vi "Initialize.vi"(8 "error in":errorcluster, 11 "Plugin in":refnum<class "Sift Stream.lvclass">) -> (0 "error out":errorcluster, 3 "Plugin out":refnum<class "Sift Stream.lvclass">)   [LabVIEW 2024, in "Sift Stream.lvlib" / "Sift Stream.lvclass"]
uses:
  Sift Stream.lvclass
  Sift Stream.lvclass/Sift Stream.ctl
  <vilib>/FlexLogger/SDK/PluginSDK.lvlibp/PEFClasses/SDK/Plugin/Plugin.lvclass
  <vilib>/FlexLogger/SDK/PluginSDK.lvlibp/PEFClasses/SDK/Processing Element/Timing Method.ctl
  <vilib>/FlexLogger/SDK/PluginSDK.lvlibp/PEFClasses/SDK/Processing Element/Processing Element.lvclass
  <vilib>/FlexLogger/SDK/PluginSDK.lvlibp/PEFClasses/SDK/Processing Element/Timing Parameters.ctl
  <vilib>/FlexLogger/SDK/PluginSDK.lvlibp/PEFClasses/SDK/Plugin/ParameterAccess/Write String.vi
  <vilib>/FlexLogger/SDK/PluginSDK.lvlibp/PEFClasses/SDK/Plugin/ParameterAccess/Write DBL.vi
  <vilib>/FlexLogger/SDK/PluginSDK.lvlibp/PEFClasses/SDK/Plugin/ParameterAccess/Write N Channel.vi
  C:/Program Files/National Instruments/LabVIEW 2024/vi.lib/FlexLogger/SDK/PluginSDK.lvlibp/PEFClasses/SDK/Plugin/Plugin.lvclass
  C:/Program Files/National Instruments/LabVIEW 2024/vi.lib/FlexLogger/SDK/PluginSDK.lvlibp/PEFClasses/SDK/Processing Element/Processing Element.lvclass
  C:/Users/Alex luCK/Documents/Projects/sift-labview/plugins/flexlogger/Sift Stream/source/Sift Stream/Sift Stream.lvclass
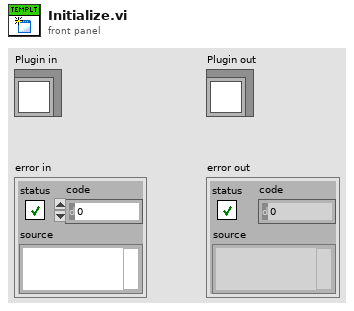
[diagram p1: front panel]
types:
  T1 = typedef "PluginSDK.lvlibp/Processing Element.lvclass/Timing Parameters.ctl" = cluster{"Timing Method":T2, "Timing Period (ms)":i32}
  T2 = typedef "PluginSDK.lvlibp/Processing Element.lvclass/Timing Method.ctl" = enum16{"Periodic", "Immediate", "On Data Ready", "Triggered"}
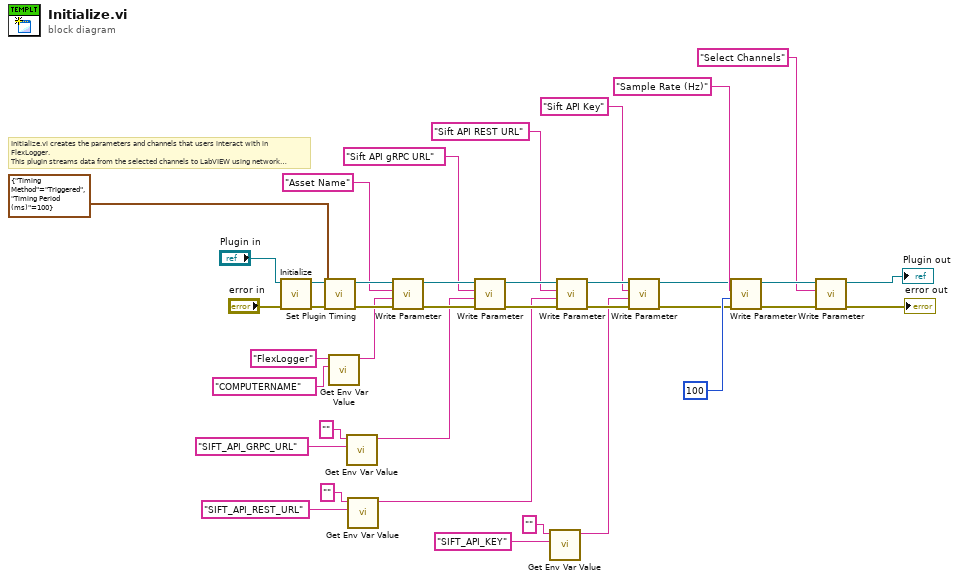
[diagram p0: block diagram]
diagram:
  # "Initialize.vi creates the parameters and channels that users interact with in FlexLogger.\nThis plugin streams data from the selected channels to LabVIEW using network streams."
  n1 = call-parent "Initialize.vi"("error in (no error)"="error in", "Plugin in"="Plugin in") -> ("error out"=w37:errorcluster, "Plugin out"=w38:refnum<class "Sift Stream.lvclass">)  [unwired: 8 in]
  n2 = call <vilib>:"Set Plugin Timing.vi"("error in (no error)"=w37, "Timing Parameters"=T1 {"Timing Method"=enum."Triggered", "Timing Period (ms)"=100}, "Plugin in"=w38) -> ("error out"=w30:errorcluster, "Plugin out"=w31:refnum<class "Sift Stream.lvclass">)  [unwired: 7 in]
  n3 = call "Get Env Var Value.vi"("env var name"="COMPUTERNAME", "default value"="FlexLogger") -> ("result"=w4:string)  [unwired: 9 in]
  n4 = call "Get Env Var Value.vi"("env var name"="SIFT_API_GRPC_URL", "default value"="") -> ("result"=w21:string)  [unwired: 9 in]
  n5 = call "Get Env Var Value.vi"("env var name"="SIFT_API_REST_URL", "default value"="") -> ("result"=w1:string)  [unwired: 9 in]
  n6 = call-poly <vilib>:"Write Parameter.vi"("error in (no error)"=w30, "Value"=w4, "Name"="Asset Name", "Plugin in"=w31) -> ("error out"=w28:errorcluster, "Plugin out"=w29:refnum<class "Sift Stream.lvclass">)  [unwired: 6 in]
  n7 = call-poly <vilib>:"Write Parameter.vi"("error in (no error)"=w28, "Value"=w21, "Name"="Sift API gRPC URL", "Plugin in"=w29) -> ("error out"=w26:errorcluster, "Plugin out"=w27:refnum<class "Sift Stream.lvclass">)  [unwired: 6 in]
  n8 = call "Get Env Var Value.vi"("env var name"="SIFT_API_KEY", "default value"="") -> ("result"=w7:string)  [unwired: 9 in]
  n9 = call-poly <vilib>:"Write Parameter.vi"("error in (no error)"=w26, "Value"=w1, "Name"="Sift API REST URL", "Plugin in"=w27) -> ("error out"=w10:errorcluster, "Plugin out"=w12:refnum<class "Sift Stream.lvclass">)  [unwired: 6 in]
  n10 = call-poly <vilib>:"Write Parameter.vi"("error in (no error)"=w10, "Value"=w7, "Name"="Sift API Key", "Plugin in"=w12) -> ("error out"=w9:errorcluster, "Plugin out"=w11:refnum<class "Sift Stream.lvclass">)  [unwired: 6 in]
  n11 = call-poly <vilib>:"Write Parameter.vi"("error in (no error)"=w9, "Value"=100, "Name"="Sample Rate (Hz)", "Plugin in"=w11) -> ("error out"=w19:errorcluster, "Plugin out"=w20:refnum<class "Sift Stream.lvclass">)  [unwired: 6 in]
  n12 = call-poly <vilib>:"Write Parameter.vi"("error in (no error)"=w19, "Name (Unique Channel Identifier)"="Select Channels", "Plugin in"=w20) -> ("error out"=→"error out":errorcluster, "Plugin out"=→"Plugin out":refnum<class "Sift Stream.lvclass">)  [unwired: 7 in]
